vi "EQC LoadFile report.vi"(11 "report file path":path) -> (0 "Error tick":bool, 2 "report (1D lines)":string[](array[string]))   [LabVIEW 2015, in "VIPM2.lvlib"]
uses:
  VIPM2.lvlib
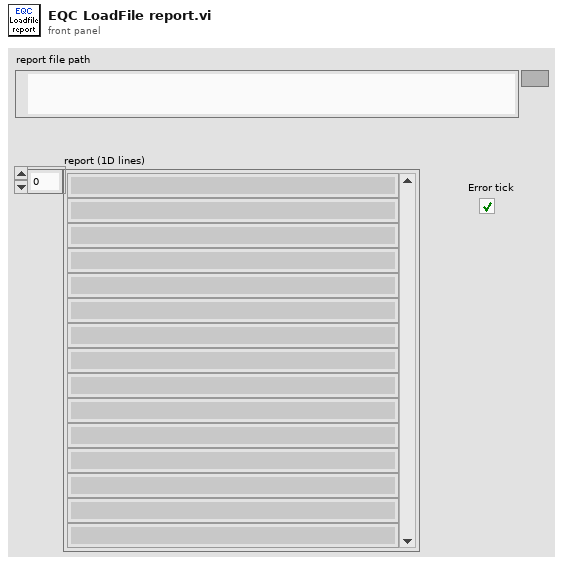
[diagram p1: front panel]
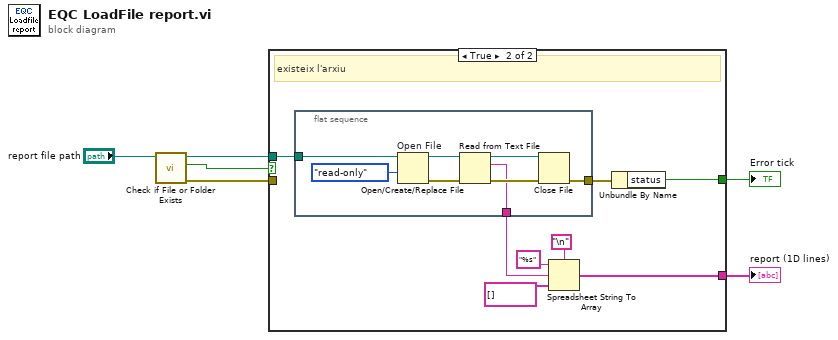
[diagram p0: block diagram]
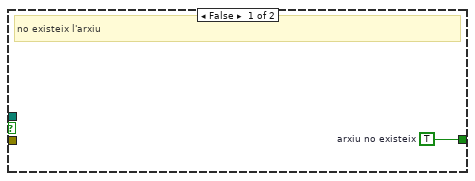
[diagram p2: hidden frame]
diagram:
  n1 = call <vilib>:"Check if File or Folder Exists.vi"("path"="report file path") -> ("error out"=w3:errorcluster, "file or folder exists?"=w2:bool, "dup path"=w5:path)  [unwired: 8 in]
  n2 = case shown="True" w2 {
    tunnel: [w7 w13] -> w6
    tunnel: w5 -> [_ w15]
    tunnel: w3 -> [_ _]
    tunnel: [_ w8] -> w1
    frame False {
      w7 = TRUE  # arxiu no existeix
      # "no existeix l'arxiu"
    }
    frame True {
      # "existeix l'arxiu"
      n3 = flat-sequence {
        tunnel: [w18] -> w14
        tunnel: w15 -> [w17]
        tunnel: [w16] -> w12
        frame #0 {
          n4 = Open/Create/Replace File "Open File"(file path (use dialog)=w17, access (0:read/write)=enum16{"read/write", "read-only", "write-only"}."read-only") -> (refnum out=w22:refnum<file>, error out=w23:errorcluster)  [unwired: 4 in, 1 out]
          n5 = Read from Text File(file (use dialog)=w22, error in=w23) -> (refnum out=w19:refnum<file>, text=w16:string, error out=w20:errorcluster)  [unwired: 2 in, 1 out]
          n6 = Close File(refnum=w19, error in=w20) -> (error out=w18:errorcluster)  [unwired: 1 out]
        }
      }
      n7 = Spreadsheet String To Array(delimiter (Tab)="\n", format string="%s", spreadsheet string=w12, array type (2D Dbl)=string[] []) -> (array=w8:string[])
      n8 = Unbundle By Name(w14) -> ("status"=w13:bool)
    }
  }
  "Error tick" <- w6
  "report (1D lines)" <- w1
